vi "PH_SHS_Analysis_Calibrator.write Pic.vi"(0 "i ref in":refnum<vi>, 2 "Cam Image":T1, 5 "error in (no error)":errorcluster) -> (14 "i ref out":refnum<vi>, 19 "error out":errorcluster)   [LabVIEW 2014, in "PH_SHS_Analysis_Calibrator.lvlib"]
doc: "This VI adds the incoming Cam Image to the background image and sets the number of accumulated pics up by one."
uses:
  PH_SHS_Analysis_Calibrator.lvlib
  <vilib>/vision/Image Controls.llb/IMAQ Image.ctl
  CS_Core/BaseSM/BaseSM.lvlib
  <vilib>/vision/NI_Vision_Development_Module.lvlib
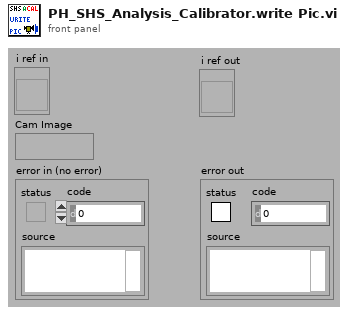
[diagram p1: front panel]
types:
  T1 = typedef "IMAQ Image.ctl" = refnum<image>
  T2 = typedef "PH_SHS_Analysis_Calibrator.lvlib/PH_SHS_Analysis_Calibrator.i attribute.ctl" = cluster{"GUI Refs":cluster{"Available Cams":refnum<vi>, "OK":refnum<vi>, "Skip":refnum<vi>, "Repeat":refnum<vi>, "Cancel":refnum<vi>, "Dialog":refnum<vi>, "Enough Images?":refnum<vi>}, "Cam instances":string[], "Status":cluster{"#":i32, "Data calculated":bool, "Wanted #":i32}, "IMAQ Image Array":T1[], "Pixel Size [µm]":dbl, "MLA Pitch [µm]":dbl, "Method":enum16{"automatic", "manual"}, "Enough Images?":bool, "SHS Reference Result":T3, "Calculation Error":errorcluster}
  T3 = typedef "SHS_Common.lvlib/SHSReference.ctl" = cluster{"Reference":T4[][], "Lens Array Pitch [px]":dbl}
  T4 = typedef "SHS_Common.lvlib/ReferencePoint.ctl" = cluster{"Rect":T5, "Point":T6}
  T5 = typedef "SHS_Common.lvlib/Rectangle.ctl" = cluster{"Left":i32, "Top":i32, "Right":i32, "Bottom":i32}
  T6 = typedef "SHS_Common.lvlib/Point.ctl" = cluster{"x":dbl, "y":dbl, "valid?":bool, "weight":dbl}
  T7 = typedef "Image Type" = u32
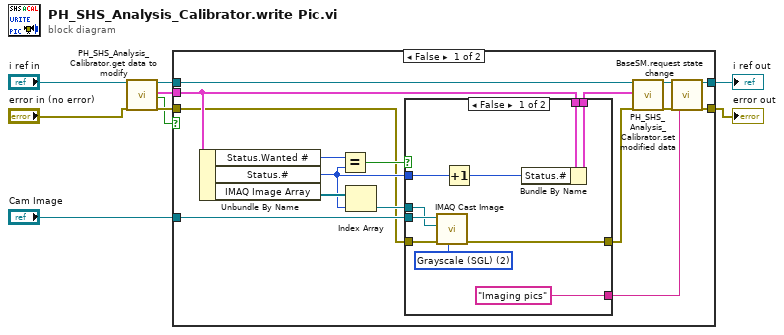
[diagram p0: block diagram]
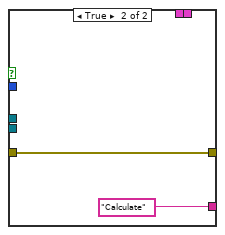
[diagram p2: hidden frame]
diagram:
  n1 = call "PH_SHS_Analysis_Calibrator.get data to modify.vi"("i ref in"="i ref in", "error in (no error)"="error in (no error)") -> ("i ref out"=w6:refnum<vi>, "i attribute"=w9:T2, "timed out"=w2:bool, "error out"=w3:errorcluster)  [unwired: 14 in]
  n2 = case shown="False" w2 {
    tunnel: "Cam Image" -> [w24 _]
    tunnel: w9 -> [w25 _]
    tunnel: [w21 w40] -> w8
    tunnel: w6 -> [w10 w40]
    tunnel: [w19 w39] -> w4
    tunnel: w3 -> [w11 w39]
    frame False {
      n3 = Unbundle By Name(w25) -> ("Status.Wanted #"=w12:i32, "Status.#"=w13:i32, "IMAQ Image Array"=w14:T1[])
      n4 = Equal?(x=w12, y=w13) -> (x = y?=w23:bool)
      n5 = Index Array(array=w14, index=w13) -> (element=w15:T1)
      n6 = case shown="False" w23 {
        tunnel: w25 -> [w33 w36]
        tunnel: w24 -> [w35 _]
        tunnel: w13 -> [w31 _]
        tunnel: ["Imaging pics" "Calculate"] -> w18
        tunnel: w15 -> [w30 _]
        tunnel: [w29 w37] -> w17
        tunnel: w11 -> [w28 w37]
        tunnel: [w27 w36] -> w16
        frame False {
          w26 = T7 2 items=["Grayscale (U8)", "Grayscale (I16)", "Grayscale (SGL)", "Complex (CSG)", "RGB (U32)", "HSL (U32)", "RGB (U64)"] ("Image Type")
          n7 = call "IMAQ Cast Image"("Image Type"=w26, "error in (no error)"=w28, "Image Dst"=w30, "Image Src"=w35) -> ("error out"=w29:errorcluster)  [unwired: 6 in, 1 out]
          n8 = Increment(x=w31) -> (x+1=w32:i32)
          n9 = Bundle By Name(cluster=w33, "Status.#"=w32) -> (w27:T2)
        }
        frame True {
        }
      }
      n10 = call "PH_SHS_Analysis_Calibrator.set modified data.vi"("i ref in"=w10, "i attribute"=w16, "error in (no error)"=w17) -> ("i ref out"=w22:refnum<vi>, "error out"=w20:errorcluster)  [unwired: 15 in]
      n11 = call "BaseSM.request state change.vi"("i ref in"=w22, "error in (no error)"=w20, "requested state"=w18) -> ("i ref out"=w21:refnum<vi>, "error out"=w19:errorcluster)  [unwired: 13 in, 2 out]
    }
    frame True {
    }
  }
  "i ref out" <- w8
  "error out" <- w4
